vi "lvapt-daily-build.vi"(11 "CommandLine":string[](array[string])) -> (2 "test details":string, 3 "exit code":i32)   [LabVIEW 2019]
panel:
  out "error out":errorcluster
  in  "error in (no error)":errorcluster
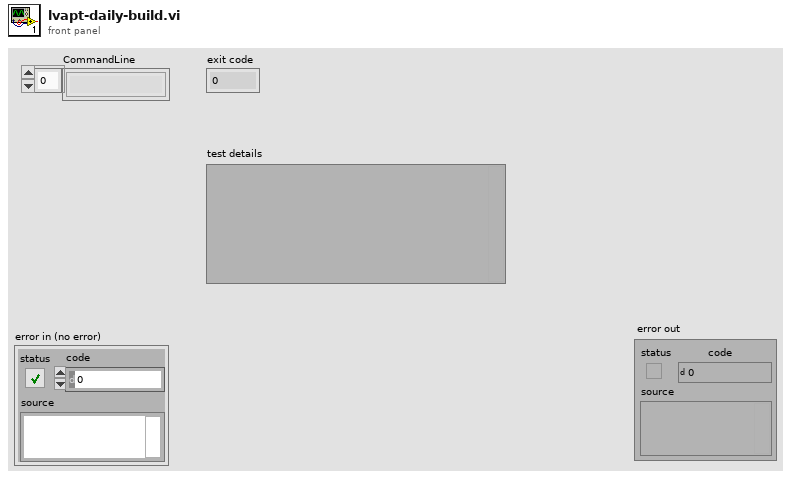
[diagram p1: front panel]
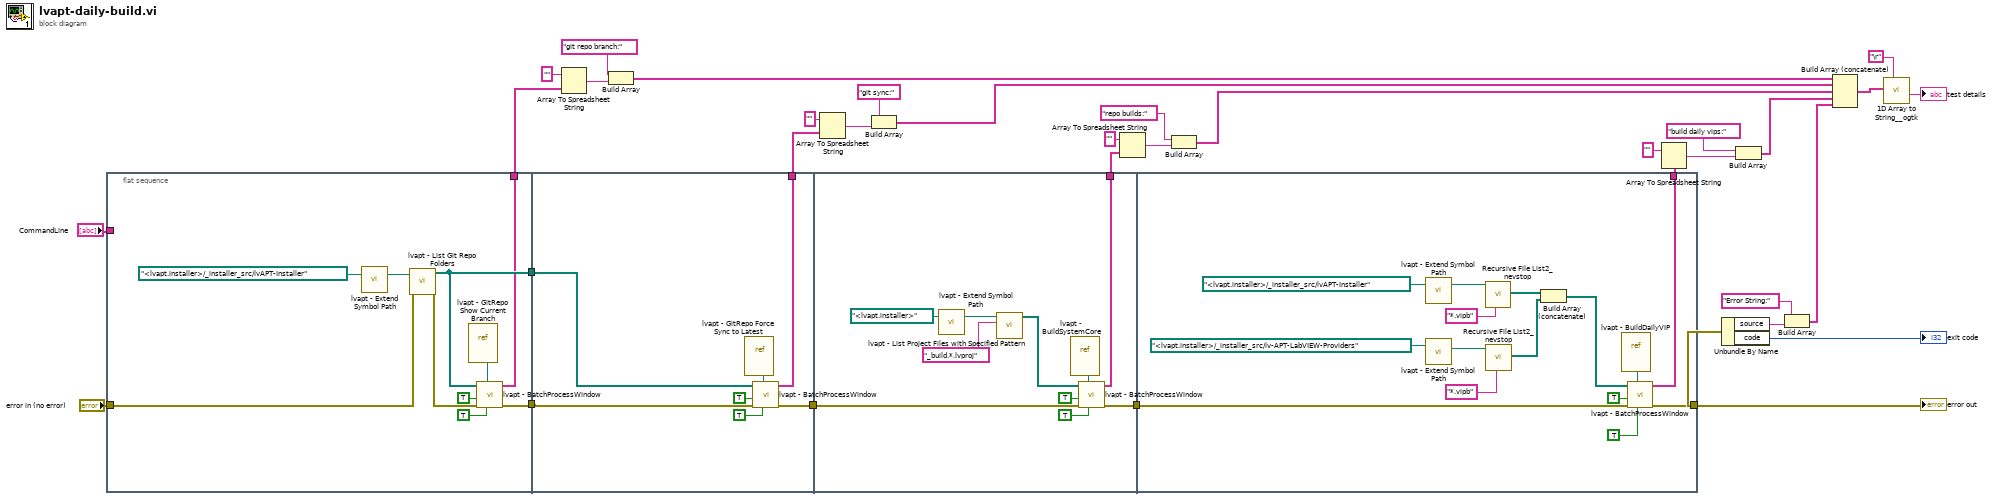
[diagram p0: block diagram]
diagram:
  n1 = flat-sequence {
    tunnel: "error in (no error)" -> [w38]
    tunnel: [w37] -> w33
    tunnel: [w36] -> w32
    tunnel: "CommandLine" -> [_]
    tunnel: [w35] -> w28
    tunnel: w33 -> [w48]
    tunnel: w32 -> [w47]
    tunnel: [w46] -> w7
    tunnel: [w45] -> w27
    tunnel: w7 -> [w58]
    tunnel: [w57] -> w6
    tunnel: [w52] -> w2
    tunnel: [w63] -> w30
    tunnel: [w62] -> w26
    tunnel: w6 -> [w64]
    frame #0 {
      n2 = call <userlib>:"lvapt - Extend Symbol Path.vi"("Symbol Path"=path "<lvapt.installer>/_installer_src/lvAPT-Installer") -> ("Resolved Path"=w40:path)  [unwired: 2 in]
      n3 = call <userlib>:"lvapt - List Git Repo Folders.vi"("error in (no error)"=w38, "path"=w40) -> ("error out"=w39:errorcluster, "Repo Folders"=w36:path[])  [unwired: 8 in]
      n4 = vi-ref <userlib>:"lvapt - GitRepo Show Current Branch.vi"() -> (w41:refnum<vi>)
      n5 = call <userlib>:"lvapt - BatchProcessWindow.vi"("FP(T)"=TRUE, "VI Refnum"=w41, "error in (no error)"=w39, "silence mode(F)"=TRUE, "paths"=w36) -> ("error out"=w37:errorcluster, "Array"=w35:string[][])  [unwired: 5 in]
    }
    frame #1 {
      n6 = vi-ref <userlib>:"lvapt - GitRepo Force Sync to Latest.vi"() -> (w51:refnum<vi>)
      n7 = call <userlib>:"lvapt - BatchProcessWindow.vi"("FP(T)"=TRUE, "VI Refnum"=w51, "error in (no error)"=w48, "silence mode(F)"=TRUE, "paths"=w47) -> ("error out"=w46:errorcluster, "Array"=w45:string[][])  [unwired: 5 in]
    }
    frame #2 {
      n8 = call <userlib>:"lvapt - Extend Symbol Path.vi"("Symbol Path"=path "<lvapt.installer>") -> ("Resolved Path"=w54:path)  [unwired: 2 in]
      n9 = call <userlib>:"lvapt - List Project Files with Specified Pattern.vi"("pattern"="_build.*.lvproj", "Path"=w54) -> ("All Files in Dir"=w53:path[])  [unwired: 7 in, 2 out]
      n10 = vi-ref <userlib>:"lvapt - BuildSystemCore.vi"() -> (w59:refnum<vi>)
      n11 = call <userlib>:"lvapt - BatchProcessWindow.vi"("FP(T)"=TRUE, "VI Refnum"=w59, "error in (no error)"=w58, "silence mode(F)"=TRUE, "paths"=w53) -> ("error out"=w57:errorcluster, "Array"=w52:string[][])  [unwired: 5 in]
    }
    frame #3 {
      n12 = call <userlib>:"lvapt - Extend Symbol Path.vi"("Symbol Path"=path "<lvapt.installer>/_installer_src/lvAPT-Installer") -> ("Resolved Path"=w72:path)  [unwired: 2 in]
      n13 = call <userlib>:"lvapt - Extend Symbol Path.vi"("Symbol Path"=path "<lvapt.installer>/_installer_src/lv-APT-LabVIEW-Providers") -> ("Resolved Path"=w71:path)  [unwired: 2 in]
      n14 = call <userlib>:"Recursive File List2_nevstop.vi"("pattern"="*.vipb", "Folder Path"=w72) -> ("All Files in Dir"=w73:path[])  [unwired: 5 in, 4 out]
      n15 = call <userlib>:"Recursive File List2_nevstop.vi"("pattern"="*.vipb", "Folder Path"=w71) -> ("All Files in Dir"=w74:path[])  [unwired: 5 in, 4 out]
      n16 = Build Array (concatenate)(w73, w74) -> (w75:path[])
      n17 = vi-ref <userlib>:"lvapt - BuildDailyVIP.vi"() -> (w76:refnum<vi>)
      n18 = call <userlib>:"lvapt - BatchProcessWindow.vi"("FP(T)"=TRUE, "VI Refnum"=w76, "error in (no error)"=w64, "silence mode(F)"=TRUE, "paths"=w75) -> ("error out"=w63:errorcluster, "Array"=w62:string[][])  [unwired: 5 in]
    }
  }
  n19 = Array To Spreadsheet String(array=w28, 3:"" ("format string")) -> (spreadsheet string=w25:string)  [unwired: 1 in]
  n20 = Build Array("git repo branch:" ("element"), w25) -> (w24:string[])
  n21 = Array To Spreadsheet String(array=w27, 3:"" ("format string")) -> (spreadsheet string=w22:string)  [unwired: 1 in]
  n22 = Build Array("git sync:" ("element"), w22) -> (w20:string[])
  n23 = Array To Spreadsheet String(array=w2, 3:"" ("format string")) -> (spreadsheet string=w3:string)  [unwired: 1 in]
  n24 = Build Array("repo builds:" ("element"), w3) -> (w1:string[])
  n25 = Array To Spreadsheet String(array=w26, 3:"" ("format string")) -> (spreadsheet string=w19:string)  [unwired: 1 in]
  n26 = Unbundle By Name(w30) -> ("source"=w16:string, "code"=→"exit code":i32)
  n27 = Build Array("build daily vips:" ("element"), w19) -> (w18:string[])
  n28 = Build Array("Error String:" ("element"), w16) -> (w14:string[])
  n29 = Build Array (concatenate)(w24, w20, w1, w18, w14) -> (w13:string[])
  n30 = call <userlib>:"1D Array to String__ogtk.vi"("delimiter (Tab)"="\r", "Array of Strings"=w13) -> ("delimited string"=→"test details":string)  [unwired: 9 in]
  "error out" <- w30
